vi "Calculate Limit Test Report.vi"(0 "Instrument Handle In":i32, 5 "Calculation Channel":i32(ring) items=["Calc Channel 1", "Calc Channel 2", "Calc Channel 3", "Calc Channel 4"], 11 "error in":errorcluster) -> (2 "Last":dbl, 3 "std_dev":dbl caption="Standard Deviation", 4 "Instrument Handle Out":i32, 6 "Count":u32, 8 "Fail":u32, 10 "Min":dbl, 13 "Average":dbl, 14 "Max":dbl, 15 "error out":errorcluster)   [LabVIEW 8.6, in "ZTScopeM.lvlib"]
doc: "Query all the limit test report data."
uses:
  ZTScopeM.lvlib
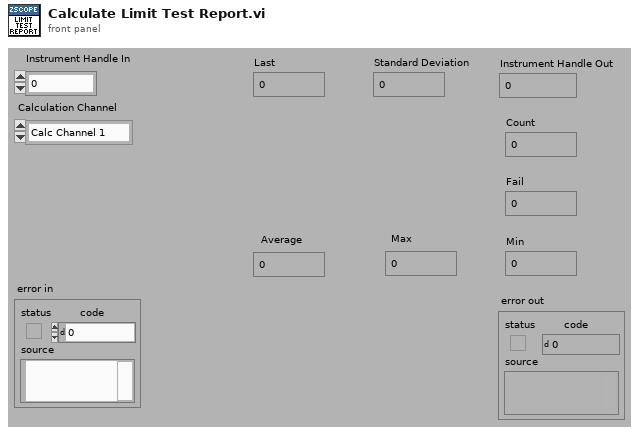
[diagram p1: front panel]
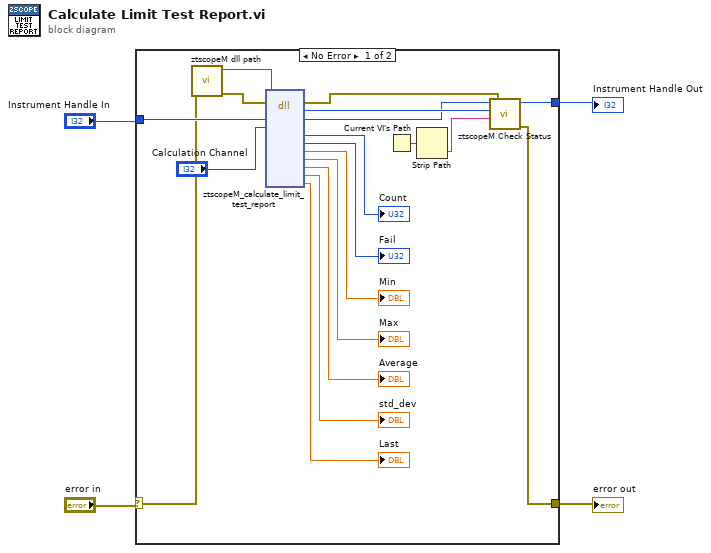
[diagram p0: block diagram]
diagram:
  n1 = case shown="No Error" "error in" {
    selector: "error in" -> [w8 w25]
    tunnel: [w10 w25] -> w1
    tunnel: "Instrument Handle In" -> [w23 w24]
    tunnel: [w9 w24] -> w3
    frame #0 {
      n2 = call "ztscopeM dll path.vi"("error in (no error)"=w8) -> ("error out"=w6:errorcluster, "<instrument>.dll path"=w7:path)  [unwired: 9 in]
      n3 = dll-call lib="C:/Program Files (x86)/National Instruments/LabVIEW 2013/instr.lib/ztscopem/ztscopeM.dll" fn="ztscopeM_calculate_limit_test_report"(path in=w7, error in=w6, "instrumentHandle"=w23, "calculationChannel"="Calculation Channel") -> (error out=w5:errorcluster, w12:i32, "instrumentHandle"=w11:i32, "count"=→"Count":u32, "failures"=→"Fail":u32, "minimum"=→"Min":dbl, "maximum"=→"Max":dbl, "average"=→"Average":dbl, "standardDeviation"=→"std_dev":dbl, "last"=→"Last":dbl)  [unwired: 9 in, 1 out]
      n4 = Current VI's Path() -> (path=w14:path)
      n5 = Strip Path(path=w14) -> (name=w13:string)  [unwired: 1 out]
      n6 = call "ztscopeM Check Status.vi"("error in"=w5, "name of VI"=w13, "status (return code)"=w12, "instrument handle in"=w11) -> ("error out"=w10:errorcluster, "instrument handle out"=w9:i32)  [unwired: 2 in]
    }
    frame #1 {
    }
  }
  "Instrument Handle Out" <- w3
  "error out" <- w1
